vi "XW_Angle_Speed_Tweak_PN.vi"(4 "Psi changes with U?":bool=TRUE, 5 "Coeffs":dbl[](array[numeric]), 6 "U1":dbl, 7 "C2":dbl, 8 "C1":dbl, 9 "C0":dbl, 10 "U2":dbl) -> (0 "V":dbl, 1 "U":dbl, 2 "Psi2 (deg)":dbl, 3 "Psi1 (deg)":dbl)   [LabVIEW 2010]
panel:
  out "abs rel. err. 2":dbl format="%#_2e"
  out "abs rel. err.1":dbl format="%#_2e"
  out "Iterations":i32
  in  "max. iter":i32=1000
  in  "Psi tol.":dbl=1e-12
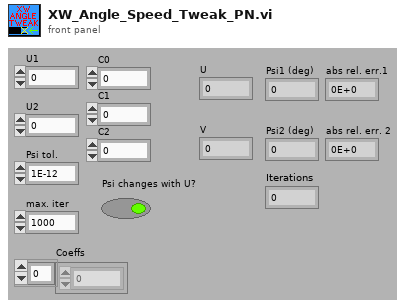
[diagram p1: front panel]
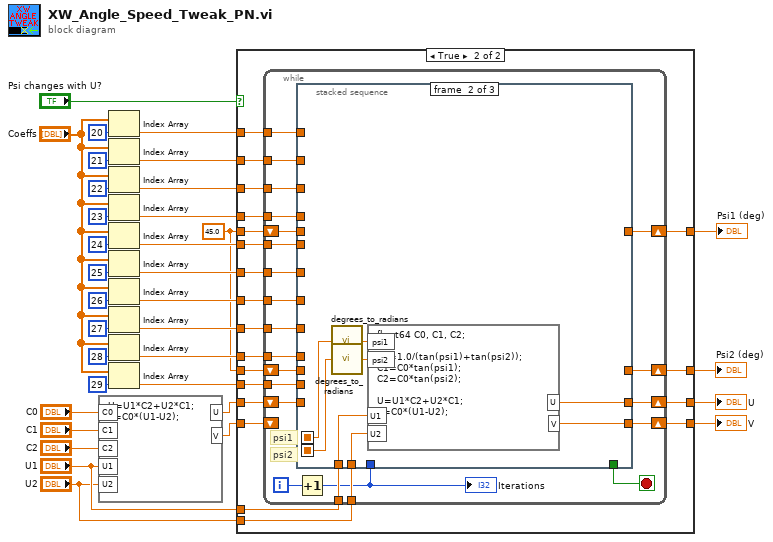
[diagram p0: block diagram]
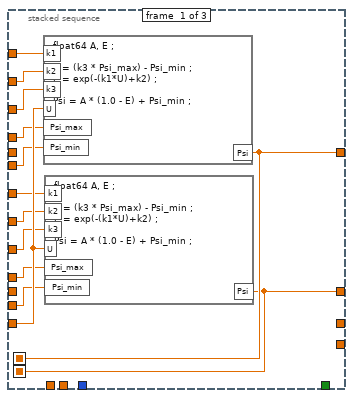
[diagram p3: hidden frame]
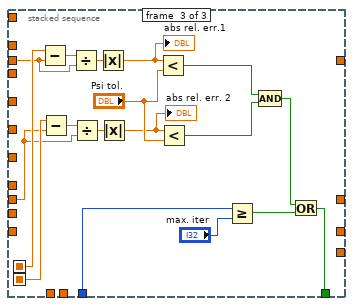
[diagram p4: hidden frame]
diagram:
  w1 = 45.0
  n1 = formula code="U=U1*C2+U2*C1;\nV=C0*(U1-U2);"("C0"="C0", "C1"="C1", "U1"="U1", "U2"="U2", "C2"="C2") -> ("U"=w33:dbl, "V"=w32:dbl)
  n2 = Index Array(array="Coeffs", index=20) -> (element=w27:dbl)
  n3 = Index Array(array="Coeffs", index=21) -> (element=w26:dbl)
  n4 = Index Array(array="Coeffs", index=22) -> (element=w24:dbl)
  n5 = Index Array(array="Coeffs", index=23) -> (element=w20:dbl)
  n6 = Index Array(array="Coeffs", index=24) -> (element=w19:dbl)
  n7 = Index Array(array="Coeffs", index=25) -> (element=w18:dbl)
  n8 = Index Array(array="Coeffs", index=26) -> (element=w16:dbl)
  n9 = Index Array(array="Coeffs", index=27) -> (element=w15:dbl)
  n10 = Index Array(array="Coeffs", index=28) -> (element=w10:dbl)
  n11 = Index Array(array="Coeffs", index=29) -> (element=w9:dbl)
  n12 = case shown="True" "Psi changes with U?" {
    tunnel: w33 -> [w38 w52]
    tunnel: w32 -> [w37 w43]
    tunnel: [w38 w42] -> w29
    tunnel: [w37 w41] -> w28
    tunnel: w27 -> [_ w58]
    tunnel: w26 -> [_ w57]
    tunnel: w24 -> [_ w56]
    tunnel: w20 -> [_ w55]
    tunnel: w19 -> [_ w54]
    tunnel: w18 -> [_ w53]
    tunnel: w16 -> [_ w51]
    tunnel: w15 -> [_ w50]
    tunnel: w10 -> [_ w49]
    tunnel: w9 -> [_ w48]
    tunnel: "U1" -> [_ w47]
    tunnel: "U2" -> [_ w46]
    tunnel: w1 -> [w36 w45]
    tunnel: w1 -> [w35 w44]
    tunnel: [w36 w40] -> w6
    tunnel: [w35 w39] -> w5
    frame False {
    }
    frame True {
      n13 = while {
        tunnel: w58 -> [w79]
        tunnel: w57 -> [w78]
        tunnel: w56 -> [w77]
        tunnel: w55 -> [w76]
        tunnel: w54 -> [w75]
        tunnel: w53 -> [w70]
        tunnel: w51 -> [w71]
        tunnel: w50 -> [w72]
        tunnel: w49 -> [w74]
        tunnel: w48 -> [w73]
        shift-right: [w69] -> w40
        shift-left: w45 -> [w63]
        shift-right: [w68] -> w39
        shift-left: w44 -> [w62]
        tunnel: w47 -> [w67]
        tunnel: w46 -> [w66]
        shift-right: [w61] -> w42
        shift-left: w52 -> [w80]
        shift-right: [w60] -> w41
        shift-left: w43 -> [_]
        i -> [w64]
        stop <- w65 stop-if-true
        # "psi2"
        # "psi1"
        n14 = Increment(x=w64) -> (x+1=w59:i32)
        "Iterations" <- w59
        n15 = stacked-sequence {
          seq-local: [w82 _ _] -> [_ w99 w113]
          seq-local: [w81 _ _] -> [_ w98 w103]
          tunnel: w80 -> [w93 _ _]
          tunnel: w79 -> [w92 _ _]
          tunnel: w78 -> [w91 _ _]
          tunnel: w77 -> [w90 _ _]
          tunnel: w76 -> [w89 _ _]
          tunnel: w75 -> [w88 _ _]
          tunnel: w74 -> [w84 _ _]
          tunnel: w73 -> [w83 _ _]
          tunnel: w72 -> [w85 _ _]
          tunnel: w71 -> [w86 _ _]
          tunnel: w70 -> [w87 _ _]
          tunnel: [w82 _ _] -> w69
          tunnel: [w81 _ _] -> w68
          tunnel: w67 -> [_ w97 _]
          tunnel: w66 -> [_ w96 _]
          tunnel: [_ _ w115] -> w65
          tunnel: w59 -> [_ _ w114]
          tunnel: w63 -> [_ _ w112]
          tunnel: w62 -> [_ _ w102]
          tunnel: [_ w95 _] -> w61
          tunnel: [_ w94 _] -> w60
          frame #0 {
            n16 = formula code="float64 A, E ;\n\nA = (k3 * Psi_max) - Psi_min ;\nE = exp(-(k1*U)+k2) ;\n\nPsi = A * (1.0 - E) + Psi_min ;"("U"=w93, "k1"=w92, "k2"=w91, "k3"=w90, "Psi_max"=w89, "Psi_min"=w88) -> ("Psi"=w82:dbl)
            n17 = formula code="float64 A, E ;\n\nA = (k3 * Psi_max) - Psi_min ;\nE = exp(-(k1*U)+k2) ;\n\nPsi = A * (1.0 - E) + Psi_min ;"("U"=w93, "k1"=w87, "k2"=w86, "k3"=w85, "Psi_max"=w84, "Psi_min"=w83) -> ("Psi"=w81:dbl)
          }
          frame #1 {
            n18 = call "degrees_to_radians.vi"("degrees"=w99) -> ("radians"=w100:dbl)
            n19 = call "degrees_to_radians.vi"("degrees"=w98) -> ("radians"=w101:dbl)
            n20 = formula code="float64 C0, C1, C2;\n\nC0=1.0/(tan(psi1)+tan(psi2));\nC1=C0*tan(psi1);\nC2=C0*tan(psi2);\n\nU=U1*C2+U2*C1;\nV=C0*(U1-U2);"("psi1"=w100, "psi2"=w101, "U1"=w97, "U2"=w96) -> ("U"=w95:dbl, "V"=w94:dbl)
          }
          frame #2 {
            n21 = Subtract(x=w113, y=w112) -> (x-y=w119:dbl)
            n22 = Subtract(x=w103, y=w102) -> (x-y=w109:dbl)
            n23 = Divide(x=w119, y=w112) -> (x/y=w118:dbl)
            n24 = Divide(x=w109, y=w102) -> (x/y=w110:dbl)
            n25 = Absolute Value(x=w118) -> (abs(x)=w111:dbl)
            "abs rel. err.1" <- w111
            n26 = Absolute Value(x=w110) -> (abs(x)=w107:dbl)
            "abs rel. err. 2" <- w107
            n27 = Less?(x=w111, y="Psi tol.") -> (x < y?=w106:bool)
            n28 = Less?(x=w107, y="Psi tol.") -> (x < y?=w105:bool)
            n29 = Greater Or Equal?(x=w114, y="max. iter") -> (x >= y?=w116:bool)
            n30 = Compound Arithmetic op=AND(w106, w105) -> (w104:bool)
            n31 = Or(x=w104, y=w116) -> (x .or. y?=w115:bool)
          }
        }
      }
    }
  }
  "Psi1 (deg)" <- w6
  "Psi2 (deg)" <- w5
  "U" <- w29
  "V" <- w28
